vi "SetSerial.vi"(0 "reference in":refnum<class "Test_Base.lvclass">, 5 "SN":string, 7 "BN":string, 9 "UUT_Index":i32, 11 "error in (no error)":errorcluster) -> (4 "reference in":refnum<class "Test_Base.lvclass">, 10 "OK":bool, 15 "error out":errorcluster)   [LabVIEW 2022 SP3, in "Test_Base.lvlib" / "Test_Base.lvclass"]
uses:
  Test_Base.lvclass
  Components/TestView_Base.lvlibp/TestView_Base.lvclass
  Components/MES_Base.lvlibp/MES_Base.lvclass
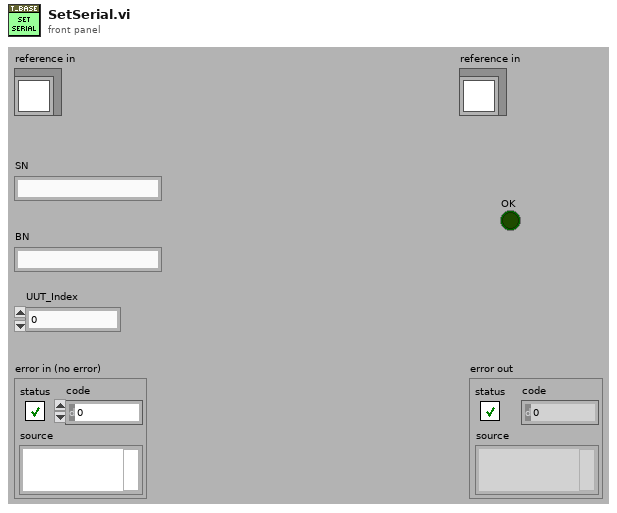
[diagram p1: front panel]
types:
  T1 = typedef "Test_Base.lvlib/Test_Base.lvclass/ObjectAttributes.ctl" = cluster{"Config":T2, "UUTIndex":i32, "Serial":string, "Batch":string, "MES":refnum<class "MES_Base.lvclass">, "TestView":refnum<class "TestView_Base.lvclass">, "LoggedIn":bool, "Abort":bool}
  T2 = typedef "Test_Base.lvlib/Test_Base.lvclass/Config.ctl" = cluster{"ContinueOnFail":bool}
  T3 = cluster{"Code":string, "Name":string, "Description":string, "Group":string, "IsGroup":bool, "Tag":string, "Method":string, "Parrameter":string, "DataType":enum16{"NA", "String", "Boolean", "Int", "Dbl"}, "Value":variant, "Status":enum16{"Pending", "Pass", "Fail"}, "LimitLo":variant, "LimitHi":variant, "StringMatch":string, "BooleanMatch":bool, "DisplayFormat":string, "Units":string, "TestTime":dbl}[]
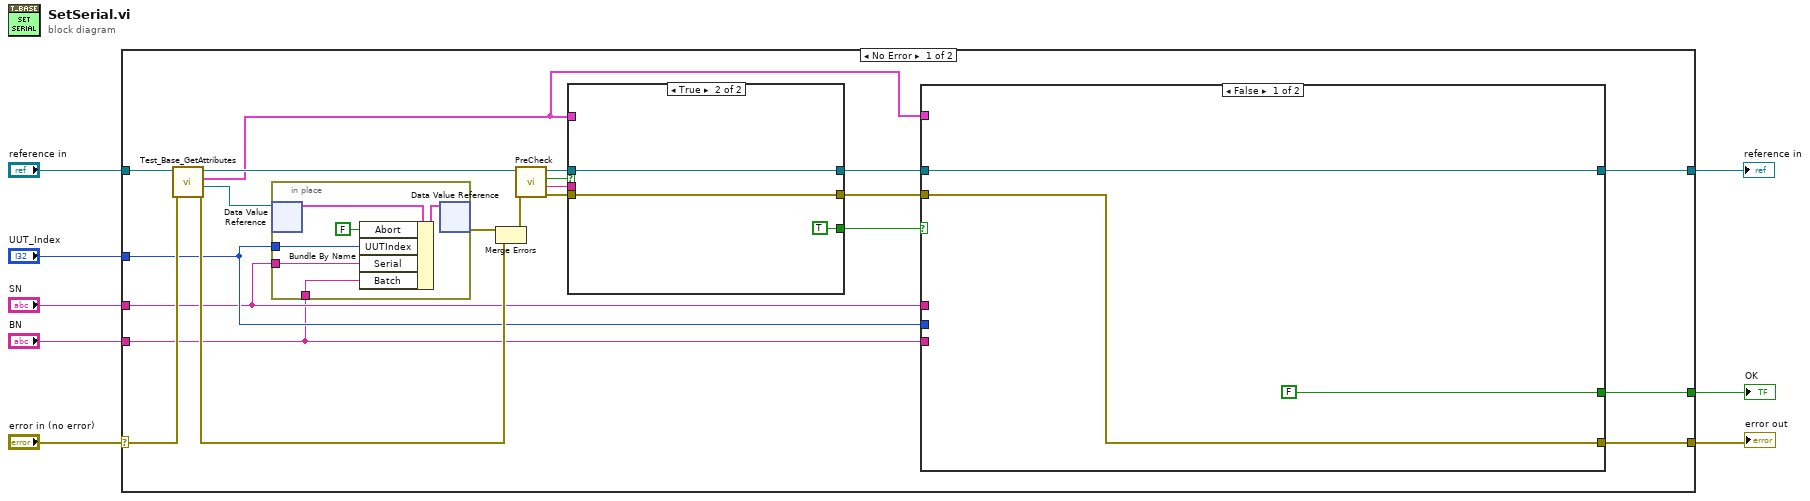
[diagram p0: block diagram]
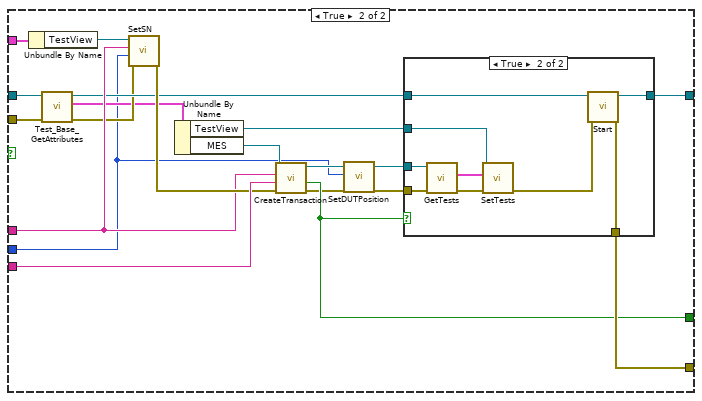
[diagram p2: hidden frame]
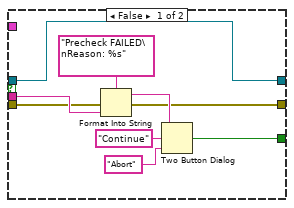
[diagram p4: hidden frame]
diagram:
  n1 = case shown="No Error" "error in (no error)" {
    selector: "error in (no error)" -> [w26 w83]
    tunnel: [w28 w83] -> w7
    tunnel: [w29 w82] -> w5
    tunnel: "reference in" -> [w27 w82]
    tunnel: "SN" -> [w10 _]
    tunnel: "BN" -> [w9 _]
    tunnel: "UUT_Index" -> [w13 _]
    tunnel: [w22 _] -> w1
    frame No Error {
      n2 = call "Test_Base_GetAttributes.vi"("error in (no error)"=w26, "reference in"=w27) -> ("error out"=w23:errorcluster, "DataRef"=w25:refnum<data-value>, "Data"=w14:T1, "reference out"=w20:refnum<class "Test_Base.lvclass">)  [unwired: 6 in]
      n3 = in-place {
        in-place-border: w13 -> [w79]
        in-place-border: w10 -> [w77]
        in-place-border: w9 -> [w76]
        n4 = in-place-dvr #1(w25) -> (w81:T1)  [unwired: 1 out]
        n5 = Bundle By Name(cluster=w81, "Abort"=FALSE, "UUTIndex"=w79, "Serial"=w77, "Batch"=w76) -> (w80:T1)
        n6 = in-place-dvr #1(w80) -> (w24:errorcluster)  [unwired: 1 out]
      }
      n7 = Merge Errors(w24, w23) -> (w21:errorcluster)
      n8 = call-dynamic "PreCheck.vi"("error in (no error)"=w21, "reference in"=w20) -> ("error out"=w19:errorcluster, "FailureMsg"=w16:string, "OK"=w18:bool, "reference in"=w17:refnum<class "Test_Base.lvclass">)  [unwired: 6 in]
      n9 = case shown="True" w18 {
        tunnel: w19 -> [w70 w74]
        tunnel: w17 -> [w64 w73]
        tunnel: w16 -> [w71 _]
        tunnel: [w66 w74] -> w11
        tunnel: [w65 TRUE ("T button?")] -> w15
        tunnel: [w64 w73] -> w12
        tunnel: w14 -> [_ _]
        frame False {
          n10 = Format Into String(format string="Precheck FAILED\nReason: %s", error in=w70, w71) -> (resulting string=w67:string, error out=w66:errorcluster)  [unwired: 1 in]
          n11 = Two Button Dialog(message=w67, 1:"Abort" ("T button name (\"OK\")"), 2:"Continue" ("T button name (\"OK\")")) -> (T button?=w65:bool)
        }
        frame True {
        }
      }
      n12 = case shown="False" w15 {
        tunnel: w10 -> [_ w43]
        tunnel: w9 -> [_ w52]
        tunnel: [w31 w51] -> w29
        tunnel: [w32 w50] -> w28
        tunnel: [FALSE ("OK") w49] -> w22
        tunnel: w11 -> [w32 w40]
        tunnel: w12 -> [w31 w42]
        tunnel: w14 -> [_ w46]
        tunnel: w13 -> [_ w33]
        frame False {
        }
        frame True {
          n13 = Unbundle By Name(w46) -> ("TestView"=w45:refnum<class "TestView_Base.lvclass">)
          n14 = call "Test_Base_GetAttributes.vi"("error in (no error)"=w40, "reference in"=w42) -> ("error out"=w39:errorcluster, "Data"=w38:T1, "reference out"=w41:refnum<class "Test_Base.lvclass">)  [unwired: 6 in, 1 out]
          n15 = call-dynamic "SetSN.vi"("error in (no error)"=w39, "DUT"=w33, "SN"=w43, "reference in"=w45) -> ("error out"=w44:errorcluster)  [unwired: 6 in, 1 out]
          n16 = Unbundle By Name(w38) -> ("TestView"=w48:refnum<class "TestView_Base.lvclass">, "MES"=w47:refnum<class "MES_Base.lvclass">)
          n17 = call-dynamic "CreateTransaction.vi"("error in (no error)"=w44, "BN"=w52, "SN"=w43, "reference in"=w47) -> ("error out"=w37:errorcluster, "OK"=w49:bool, "reference in"=w35:refnum<class "MES_Base.lvclass">)  [unwired: 4 in]
          n18 = call-dynamic "SetDUTPosition.vi"("reference in"=w35, "DUT Position"=w33, "error in (no error)"=w37) -> ("reference in"=w34:refnum<class "MES_Base.lvclass">, "error out"=w36:errorcluster)  [unwired: 15 in]
          n19 = case shown="True" w49 {
            tunnel: w41 -> [w54 w61]
            tunnel: [w54 w63] -> w51
            tunnel: [w53 w62] -> w50
            tunnel: w34 -> [_ w60]
            tunnel: w36 -> [w53 w59]
            tunnel: w48 -> [_ w58]
            frame False {
            }
            frame True {
              n20 = call-dynamic "GetTests.vi"("error in (no error)"=w59, "reference in"=w60) -> ("error out"=w57:errorcluster, "Tests"=w55:T3)  [unwired: 6 in, 2 out]
              n21 = call-dynamic "SetTests.vi"("error in (no error)"=w57, "Tests"=w55, "reference in"=w58) -> ("error out"=w56:errorcluster)  [unwired: 7 in, 1 out]
              n22 = call-dynamic "Start.vi"("error in (no error)"=w56, "reference in"=w61) -> ("error out"=w62:errorcluster, "reference in"=w63:refnum<class "Test_Base.lvclass">)  [unwired: 8 in]
            }
          }
        }
      }
    }
    frame Error {
    }
  }
  "error out" <- w7
  "reference in" <- w5
  "OK" <- w1
